vi "HC-SR04 Get Distance.vi"(0 "Arduino Resource":T1={"VISA resource"="", "Board Type"=enum."Uno", "Connection Type"=enum."USB / Serial", "Bytes Per Packet (15)"=15}, 5 "Trigger Pin":u8, 7 "Signal Pin":u8, 11 "error in (no error)":errorcluster) -> (4 "Arduino Resource":T1={"VISA resource"="", "Board Type"=enum."Uno", "Connection Type"=enum."USB / Serial", "Bytes Per Packet (15)"=15}, 8 "Distance (cm)":dbl, 15 "error out":errorcluster)   [LabVIEW 2012, in "LIFA Ultrasonic Distance.lvlib"]
doc: "Gets the distance from the HC-SR04."
uses:
  LIFA Ultrasonic Distance.lvlib
  <vilib>/LabVIEW Interface for Arduino/Type Defs/Board Type.ctl
  <vilib>/LabVIEW Interface for Arduino/LabVIEW Interface for Arduino.lvlib
  <vilib>/LabVIEW Interface for Arduino/Type Defs/Arduino Resource.ctl
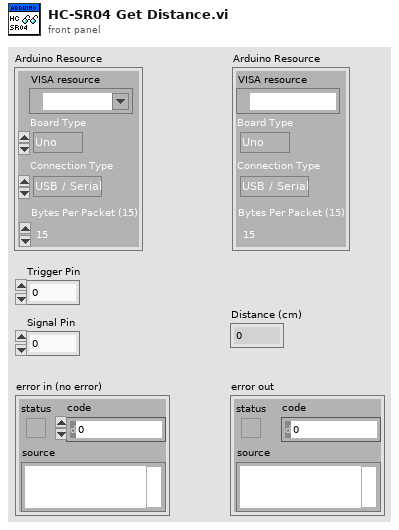
[diagram p1: front panel]
types:
  T1 = typedef "LabVIEW Interface for Arduino.lvlib/Arduino Resource.ctl" = cluster{"VISA resource":refnum<visa-resource-name>, "Board Type":T2, "Connection Type":enum8{"USB / Serial"}, "Bytes Per Packet (15)":u8}
  T2 = typedef "LabVIEW Interface for Arduino.lvlib/Board Type.ctl" = enum16{"Uno", "Dimuelanove w/Atmega 328", "Mega 2560"}
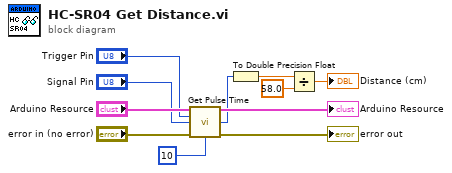
[diagram p0: block diagram]
diagram:
  n1 = call "Get Pulse Time.vi"("Arduino Resource"="Arduino Resource", "Trigger Pin"="Trigger Pin", "Signal Pin"="Signal Pin", "error in (no error)"="error in (no error)", "Trigger Length (us)"=u8 10) -> ("Arduino Resource"=→"Arduino Resource":T1, "Pulse Time (us)"=w4:u32, "error out"=→"error out":errorcluster)  [unwired: 8 in]
  n2 = To Double Precision Float(number=w4) -> (double precision float=w3:dbl)
  n3 = Divide(x=w3, y=58.0) -> (x/y=→"Distance (cm)":dbl)
